vi "Draw Gradient Rect.vi"(8 "Color Segement":u32[](array[colorbox])=[16448250, 0, 16736786, 1198079], 9 "Mode":enum16{"Horizontal", "Vertical"}(ring), 10 "rect":T1 caption="矩形", 11 "picture in":picture) -> (3 "picture out":picture)   [LabVIEW 2011]
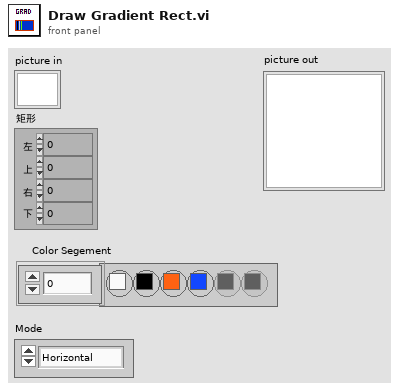
[diagram p1: front panel]
types:
  T1 = cluster{"left":i16, "top":i16, "right":i16, "bottom":i16}
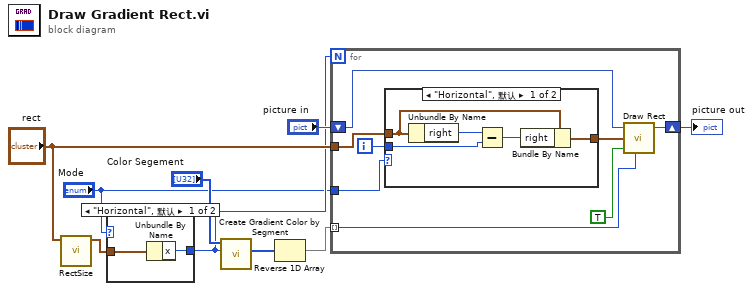
[diagram p0: block diagram]
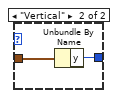
[diagram p2: hidden frame]
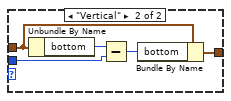
[diagram p3: hidden frame]
diagram:
  n1 = call "RectSize.vi"("rect"="rect") -> ("point"=w3:cluster{"x":i16, "y":i16})  [unwired: 7 in, 3 out]
  n2 = case shown="\"Horizontal\", 默认" "Mode" {
    tunnel: w3 -> [w11 w12]
    tunnel: [w10 w13] -> w2
    frame "Horizontal", Default {
      n3 = Unbundle By Name(w11) -> ("x"=w10:i16)
    }
    frame "Vertical" {
      n4 = Unbundle By Name(w12) -> ("y"=w13:i16)
    }
  }
  n5 = call "Create Gradient Color by Segment.vi"("Length"=w2, "Color Segement"="Color Segement") -> ("1 Pix W - Color Box Array"=w5:u32[])  [unwired: 7 in, 2 out]
  n6 = Reverse 1D Array(array=w5) -> (reversed array=w4:u32[])
  n7 = for {
    N: w2 -> [_]
    shift-right: [w20] -> w7
    shift-left: "picture in" -> [w21]
    tunnel: w4 -> [w17] mode=indexing
    tunnel: "rect" -> [w19]
    tunnel: "Mode" -> [w15]
    i -> [w16]
    n8 = case shown="\"Horizontal\", 默认" w15 {
      tunnel: w19 -> [w25 w28]
      tunnel: [w23 w27] -> w18
      tunnel: w16 -> [w22 w30]
      frame "Horizontal", Default {
        n9 = Unbundle By Name(w25) -> ("right"=w26:i16)
        n10 = Subtract(x=w26, y=w22) -> (x-y=w24:i32)
        n11 = Bundle By Name(cluster=w25, "right"=w24) -> (w23:T1)
      }
      frame "Vertical" {
        n12 = Unbundle By Name(w28) -> ("bottom"=w31:i16)
        n13 = Subtract(x=w31, y=w30) -> (x-y=w29:i32)
        n14 = Bundle By Name(cluster=w28, "bottom"=w29) -> (w27:T1)
      }
    }
    n15 = call <vilib>:"Draw Rect.vi"("picture"=w21, "rect"=w18, "fill?(F)"=TRUE, "color(black)"=w17) -> ("new picture"=w20:picture)  [unwired: 5 in]
  }
  "picture out" <- w7
